vi "Addon.Dialog.vi"(8 "error in (no error)":errorcluster) -> (0 "error out":errorcluster, 2 "Diagnostics Basic Configuraiton":T1, 3 "Cancelled?":bool)   [LabVIEW 2015, in "Diagnostics Addon System Explorer.lvlib"]
uses:
  Diagnostics Addon System Explorer.lvlib
  Shared/Types/Protocol.ctl
  Shared/Types/CAN.Interface.ctl
  Types/Addon.Initialize.ctl
  Shared/Diagnostics Addon Shared.lvlib
panel:
  in  "Path":path caption="Previous Personality Path (Optional)"
  in  "Cancel":bool
  in  "OK":bool
  in  "Baud Rate":u32=250000
  in  "CAN Interface":T2
  in  "Diagnostic Protocol":T3
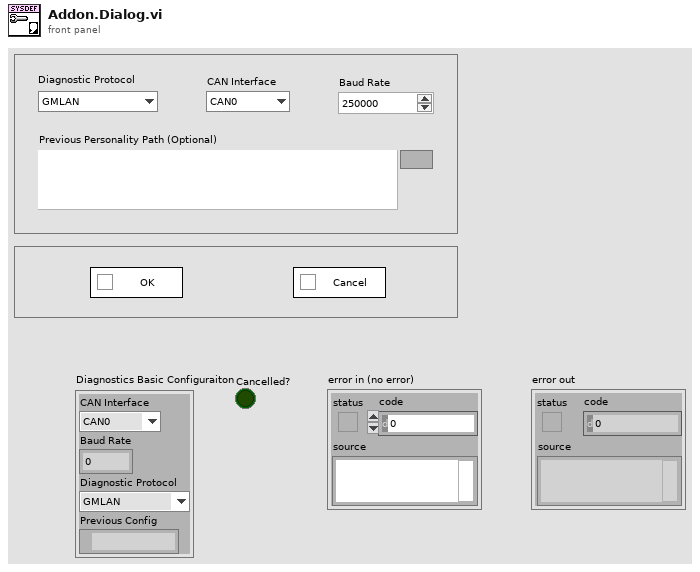
[diagram p1: front panel]
types:
  T1 = typedef "Diagnostics Addon System Explorer.lvlib/Addon.Initialize.ctl" = cluster{"CAN Interface":T2, "Baud Rate":u32, "Diagnostic Protocol":T3, "Previous Config":path}
  T2 = typedef "Diagnostics Addon Shared.lvlib/CAN.Interface.ctl" = enum16{"CAN0", "CAN1", "CAN2", "CAN3", "CAN4", "CAN5", "CAN6", "CAN7", "CAN8", "CAN9", "CAN10", "CAN11", "CAN12", "CAN13", "CAN14", "CAN15", "CAN16", "CAN17", "CAN18", "CAN19", "CAN20", "CAN21", "CAN22", "CAN23", "CAN24", "CAN25", "CAN26", "CAN27", "CAN28", "CAN29", "CAN30", "CAN31", "CAN32", "CAN33", "CAN34", "CAN35", "CAN36", "CAN37", "CAN38", "CAN39", "CAN40", "CAN41", "CAN42", "CAN43", "CAN44", "CAN45", "CAN46", "CAN47", "CAN48", "CAN49", "CAN50", "CAN51", "CAN52", "CAN53", "CAN54", "CAN55", "CAN56", "CAN57", "CAN58", "CAN59", "CAN60", "CAN61", "CAN62", "CAN63", "CAN 256 (Virtual)", "CAN 257 (Virtual)"}
  T3 = typedef "Diagnostics Addon Shared.lvlib/Protocol.ctl" = enum16{"GMLAN", "KWP-2000", "UDS", "User-Defined"}
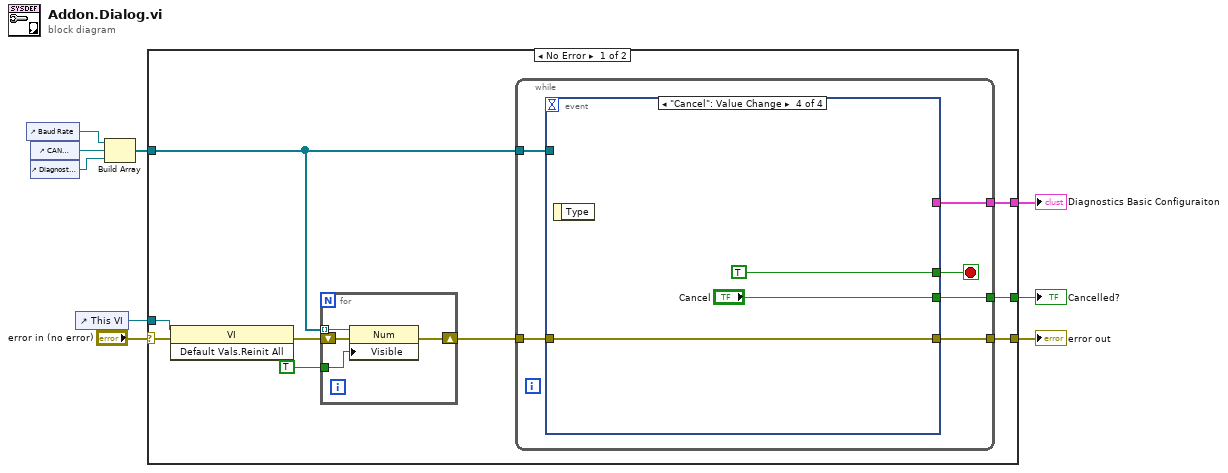
[diagram p0: block diagram]
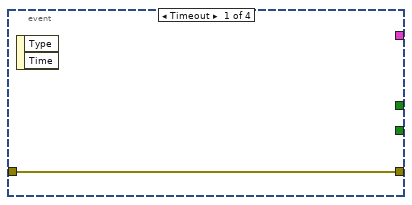
[diagram p2: hidden frame]
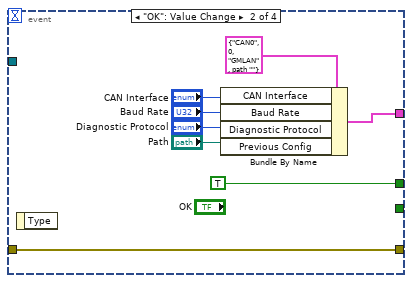
[diagram p3: hidden frame]
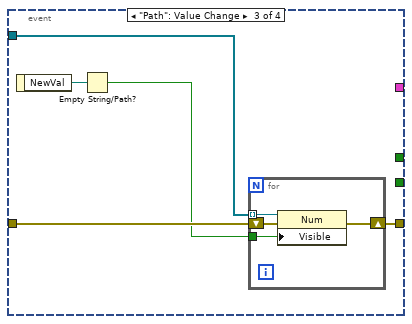
[diagram p4: hidden frame]
diagram:
  n1 = control-ref of="Baud Rate"() -> (w2:refnum<vi>)
  n2 = control-ref of="CAN Interface"() -> (w3:refnum<vi>)
  n3 = control-ref of="Diagnostic Protocol"() -> (w4:refnum<vi>)
  n4 = control-ref of="This VI"() -> (w5:refnum<vi>)
  n5 = Build Array(w2, w3, w4) -> (w1:refnum<vi>[])
  n6 = case shown="No Error" "error in (no error)" {
    selector: "error in (no error)" -> [w15 w50]
    tunnel: [w18 _] -> w9
    tunnel: [w17 _] -> w8
    tunnel: [w14 w50] -> w6
    tunnel: w5 -> [w16 _]
    tunnel: w1 -> [w11 _]
    frame No Error {
      n7 = invoke class="VI" method="Default Vals.Reinit All"(reference=w16, error in=w15) -> (error out=w13:errorcluster)  [unwired: 1 in, 2 out]
      n8 = for {
        tunnel: w11 -> [w22] mode=indexing
        shift-right: [w20] -> w12
        shift-left: w13 -> [w21]
        tunnel: TRUE -> [w19]
        n9 = property class="Num"(reference=w22, error in=w21, "Visible"=w19) -> (error out=w20:errorcluster)  [unwired: 1 out]
      }
      n10 = while {
        tunnel: [w28] -> w18
        tunnel: [w26] -> w17
        tunnel: [w24] -> w14
        tunnel: w12 -> [w25]
        tunnel: w11 -> [w23]
        stop <- w27 stop-if-true
        n11 = event shown="[3] \"Cancel\": Value Change" {
          selector: _ -> [_ _ _ _]
          dyn-events: _ -> [_ _ _ _]
          timeout: _ -> [_ _ _ _]
          tunnel: [_ _ _ "Cancel"] -> w28
          tunnel: [_ TRUE _ TRUE] -> w27
          tunnel: [_ w33 _ _] -> w26
          tunnel: w25 -> [w29 w31 w41 w47]
          tunnel: [w29 w31 w40 w47] -> w24
          tunnel: w23 -> [_ _ w39 _]
          event Timeout {
            n12 = event-data() -> ()  [unwired: 1 in, 2 out]
          }
          event "OK": Value Change {
            n13 = event-data() -> ()  [unwired: 1 in, 1 out]
            n14 = Bundle By Name(cluster=T1 {"CAN Interface"=enum."CAN0", "Baud Rate"=0, "Diagnostic Protocol"=enum."GMLAN", "Previous Config"=path ""} ("output cluster"), "CAN Interface"="CAN Interface", "Baud Rate"="Baud Rate", "Diagnostic Protocol"="Diagnostic Protocol", "Previous Config"="Path") -> (w33:T1)
          }
          event "Path": Value Change {
            n15 = event-data() -> ("NewVal"=w42:path)  [unwired: 1 in]
            n16 = Empty String/Path?(string/path=w42) -> (empty?=w38:bool)
            n17 = for {
              tunnel: w39 -> [w46] mode=indexing
              shift-right: [w44] -> w40
              shift-left: w41 -> [w45]
              tunnel: w38 -> [w43]
              n18 = property class="Num"(reference=w46, error in=w45, "Visible"=w43) -> (error out=w44:errorcluster)  [unwired: 1 out]
            }
          }
          event "Cancel": Value Change {
            n19 = event-data() -> ()  [unwired: 1 in, 1 out]
          }
        }
      }
    }
    frame Error {
    }
  }
  "Cancelled?" <- w9
  "Diagnostics Basic Configuraiton" <- w8
  "error out" <- w6
